vi "Get dBSPL from Frequency Amplitude List.vi"(0 "Semiconductor Module Context":T2, 5 "Sampling Rate":dbl format="%#_13g", 7 "Per Site Freq-Amp Data":T1[](array[typedef]), 11 "error in (no error)":errorcluster) -> (4 "Per-Site Per-FreqAmpPair dB SPL":dbl[][](array[numeric]), 15 "error out":errorcluster)   [LabVIEW 2020]
doc: "VI returns the Per-Site dB SPL value for Frequency-Amplitude List passed by user under specified sampling rate."
uses:
  <vilib>/NI_TestStand_SemiconductorModule/NI_TestStand_Semiconductor_Module.lvlibp/PinMap/General/SemiconductorModuleContext.ctl
  Per Site Sweep Data.ctl
  39a3ab5d-a6ea-4647-a559-e26a8959450b.vi
  6f0c4c81-6e94-4ac5-a946-327ae8ed193a.vi
  5552eb16-1d18-42dc-8af5-180ba06daae6.vi
  39a3ab5d-a6ea-4647-a559-e26a8959450b.vi/33b32ade-f888-404a-a29a-eab858b439c4.vi
  <vilib>/measure/matone.llb/Extract Single Tone Information N Chan.vi
  <vilib>/NI_TestStand_SemiconductorModule/NI_TestStand_Semiconductor_Module.lvlibp
  <vilib>/measure/NI_MAPro.lvlib
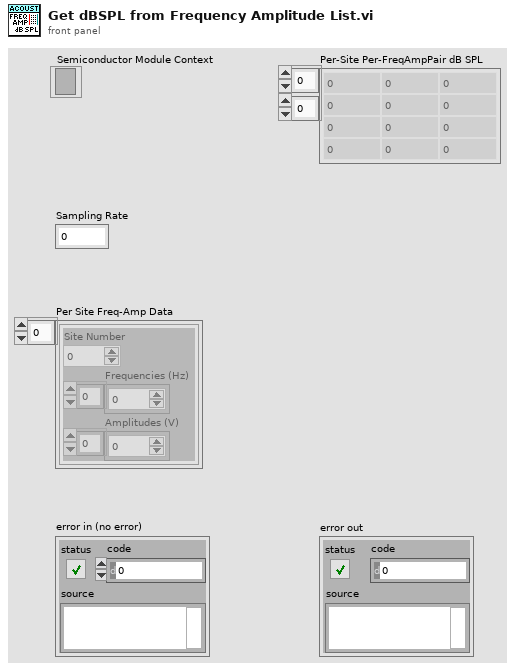
[diagram p1: front panel]
types:
  T1 = typedef "Per Site Sweep Data.ctl" = cluster{"Site Number":i32, "Frequencies (Hz)":dbl[], "Amplitudes (V)":dbl[]}
  T2 = typedef "NI_TestStand_Semiconductor_Module.lvlibp/SemiconductorModuleContext.ctl" = refnum<k7>
  T3 = typedef "TSM DAQmx Multi-Task.ctl" = cluster{"Pin Query Context":refnum<class "MultiplePinMultipleSessionQueryContext.lvclass">, "SSC":T4[], "Site Numbers":i32[], "Pins":tag[]}
  T4 = typedef "SSC DAQmx.ctl" = cluster{"DAQmx Task ":refnum<k21>, "Channels":string, "Channel Lists":string}
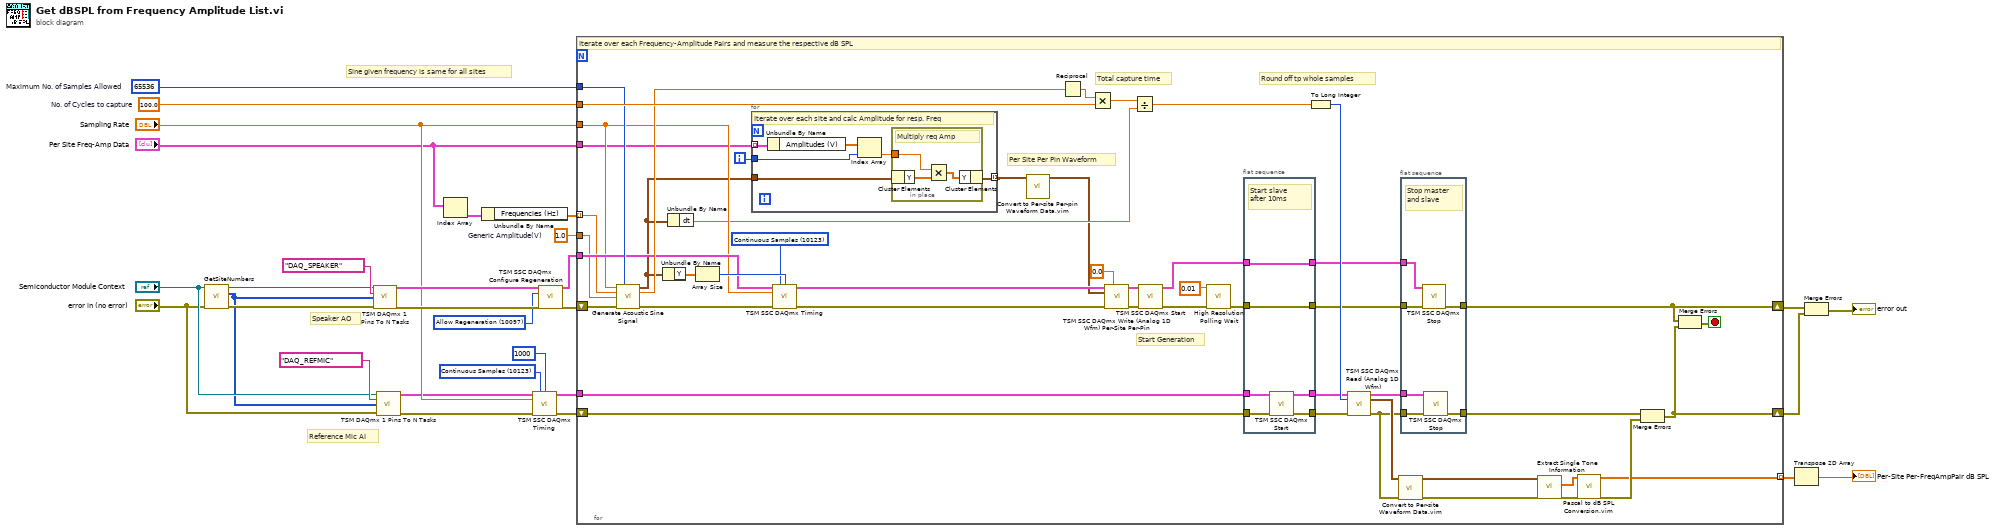
[diagram p0: block diagram]
diagram:
  w1 = 1.0  # Generic Amplitude(V)
  w11 = 65536  # Maximum No. of Samples Allowed
  w16 = 100.0  # No. of Cycles to capture
  w20 = 10123 items=["Finite Samples"=10178, "Continuous Samples"=10123, "Hardware Timed Single Point"=12522] ("Sample Mode")
  w27 = 10097 items=["Allow Regeneration"=10097, "Do Not Allow Regeneration"=10158] ("RegenMode")
  # "Sine given frequency is same for all sites"
  # "Reference Mic AI"
  # "Speaker AO"
  n1 = call <vilib>:"GetSiteNumbers.vi"("error in (no error)"="error in (no error)", "Semiconductor Module Context"="Semiconductor Module Context") -> ("error out"=w25:errorcluster, "Site Numbers"=w4:i32[], "Semiconductor Module Context Out"=w26:T2)  [unwired: 6 in, 1 out]
  n2 = call "TSM DAQmx 1 Pins To N Tasks.vi"("TSM context"=w26, "Pins"=tag "DAQ_SPEAKER", "Site Numbers"=w4, "error in"=w25) -> ("DAQ TSM Out"=w29:T3, "error out"=w30:errorcluster)  [unwired: 10 in]
  n3 = call "TSM DAQmx 1 Pins To N Tasks.vi"("TSM context"="Semiconductor Module Context", "Pins"=tag "DAQ_REFMIC", "Site Numbers"=w4, "error in"="error in (no error)") -> ("DAQ TSM Out"=w8:T3, "error out"=w9:errorcluster)  [unwired: 10 in]
  n4 = Index Array(array="Per Site Freq-Amp Data") -> (element=w3:T1)  [unwired: 1 in]
  n5 = Unbundle By Name(w3) -> ("Frequencies (Hz)"=w2:dbl[])
  n6 = call "TSM SSC DAQmx Timing.vi"("DAQ TSM in"=w8, "Sample Mode"=w20, "Samples"=1000, "Sample Rate"="Sampling Rate", "error in (no error)"=w9) -> ("DAQ TSM Out"=w19:T3, "error out"=w18:errorcluster)  [unwired: 9 in]
  n7 = call "TSM SSC DAQmx Configure Regeneration.vi"("TSM DAQmx In"=w29, "RegenMode"=w27, "error in (no error)"=w30) -> ("TSM DAQmx Out"=w24:T3, "error out"=w23:errorcluster)  [unwired: 11 in]
  n8 = for {
    shift-right: [w72] -> w15
    shift-left: w23 -> [w78]
    shift-right: [w71] -> w10
    shift-left: w18 -> [w75]
    tunnel: "Sampling Rate" -> [w62]
    tunnel: w16 -> [w77]
    tunnel: w11 -> [w76]
    tunnel: w24 -> [w64]
    tunnel: w19 -> [w74]
    tunnel: [w39] -> w7 mode=indexing
    tunnel: "Per Site Freq-Amp Data" -> [w36]
    tunnel: w2 -> [w37] mode=indexing
    tunnel: w1 -> [w38]
    i -> [w35]
    stop <- w70 stop-if-true
    w68 = 10123 items=["Finite Samples"=10178, "Continuous Samples"=10123, "Hardware Timed Single Point"=12522] ("Sample Mode")
    # "Per Site Per Pin Waveform"
    # "Start Generation"
    # "Round off tp whole samples"
    # "Total capture time"
    # "Iterate over each Frequency-Amplitude Pairs and measure the respective dB SPL"
    n9 = call "Generate Acoustic Sine Signal.vi"("Sampling Rate"=w62, "Maximum No. of Samples Allowed"=w76, "Frequency"=w37, "Sine wave amplitude"=w38, "error in (no error)"=w78) -> ("waveform"=w34:waveform(dbl), "Actual Frequency"=w73:dbl, "error out"=w67:errorcluster)  [unwired: 8 in]
    n10 = Unbundle By Name(w34) -> ("Y"=w65:dbl[])
    n11 = Unbundle By Name(w34) -> ("dt"=w44:dbl)
    n12 = Array Size(array=w65) -> (size(s)=w69:i32)
    n13 = for {
      tunnel: w36 -> [w84] mode=indexing
      tunnel: w35 -> [w82]
      tunnel: w34 -> [w81]
      tunnel: [w79] -> w33 mode=indexing
      # "Iterate over each site and calc Amplitude for resp. Freq"
      n14 = Unbundle By Name(w84) -> ("Amplitudes (V)"=w83:dbl[])
      n15 = Index Array(array=w83, index=w82) -> (element=w80:dbl)
      n16 = in-place {
        in-place-border: w80 -> [w86]
        # "Multiply req Amp"
        n17 = in-place-cluster #1(w81) -> ("Y"=w87:dbl[])
        n18 = Multiply(x=w86, y=w87) -> (x*y=w85:dbl[])
        n19 = in-place-cluster #1("Y"=w85) -> (w79:waveform(dbl))
      }
    }
    n20 = call "TSM SSC DAQmx Timing.vi"("DAQ TSM in"=w64, "Sample Mode"=w68, "Samples"=w69, "Sample Rate"=w62, "error in (no error)"=w67) -> ("DAQ TSM Out"=w63:T3, "error out"=w66:errorcluster)  [unwired: 9 in]
    n21 = call "Convert to Per-site Per-pin Waveform Data.vim"("Waveform In"=w33) -> ("Per Site Per Pin Waveform Out"=w32:waveform(dbl)[][])  [unwired: 14 in]
    n22 = Reciprocal(x=w73) -> (1/x=w43:dbl)
    n23 = Multiply(x=w43, y=w77) -> (x*y=w54:dbl)
    n24 = call "TSM SSC DAQmx Write (Analog 1D Wfm) Per-Site Per-Pin.vi"("DAQ TSM in"=w63, "Idle Channel Value (0)"=0.0, "Per-Site Per-Pin Waveforms in"=w32, "error in"=w66) -> ("DAQ TSM Out"=w61:T3, "error out"=w57:errorcluster)  [unwired: 10 in]
    n25 = Divide(x=w54, y=w44) -> (x/y=w53:dbl)
    n26 = call "TSM SSC DAQmx Start.vi"("TSM DAQmx In"=w61, "error in (no error)"=w57) -> ("TSM DAQmx Out"=w48:T3, "error out"=w55:errorcluster)  [unwired: 12 in]
    n27 = call <vilib>:"High Resolution Polling Wait.vi"("error in (no error)"=w55, "seconds to wait"=0.01) -> ("error out"=w46:errorcluster)  [unwired: 9 in]
    n28 = flat-sequence {
      tunnel: w75 -> [w93]
      tunnel: w74 -> [w92]
      tunnel: [w91] -> w50
      tunnel: [w90] -> w49
      tunnel: w48 -> [w89]
      tunnel: [w89] -> w47
      tunnel: w46 -> [w88]
      tunnel: [w88] -> w45
      frame #0 {
        # "Start slave after 10ms"
        n29 = call "TSM SSC DAQmx Start.vi"("TSM DAQmx In"=w92, "error in (no error)"=w93) -> ("TSM DAQmx Out"=w90:T3, "error out"=w91:errorcluster)  [unwired: 12 in]
      }
    }
    n30 = To Long Integer(number=w53) -> (32bit integer=w52:i32)
    n31 = call "TSM SSC DAQmx Read (Analog 1D Wfm).vi"("DAQ TSM in"=w49, "Samples to read"=w52, "error in"=w50) -> ("DAQ TSM Out"=w60:T3, "Per-Site Per-Pin Waveforms Out"=w59:waveform(dbl)[][], "error out"=w42:errorcluster)  [unwired: 10 in]
    n32 = call "Convert to Per-site Waveform Data.vim"("Per-Site Per-Pin Waveform In"=w59) -> ("Per-Site Waveform Out"=w58:waveform(dbl)[])  [unwired: 14 in]
    n33 = flat-sequence {
      tunnel: w45 -> [w99]
      tunnel: w47 -> [w98]
      tunnel: [w97] -> w72
      tunnel: w42 -> [w96]
      tunnel: [w95] -> w41
      tunnel: w60 -> [w94]
      frame #0 {
        # "Stop master and slave"
        n34 = call "TSM SSC DAQmx Stop.vi"("TSM DAQmx In"=w98, "error in (no error)"=w99) -> ("error out"=w97:errorcluster)  [unwired: 12 in, 1 out]
        n35 = call "TSM SSC DAQmx Stop.vi"("TSM DAQmx In"=w94, "error in (no error)"=w96) -> ("error out"=w95:errorcluster)  [unwired: 12 in, 1 out]
      }
    }
    n36 = call-poly <vilib>:"Extract Single Tone Information.vi"("error in (no error)"=w42, "time signals in"=w58) -> ("error out"=w40:errorcluster, "detected amplitudes"=w31:dbl[])  [unwired: 4 in, 4 out]
    n37 = call "Pascal to dB SPL Conversion.vim"("Pascals"=w31) -> ("dbSPL"=w39:dbl[])  [unwired: 14 in]
    n38 = Merge Errors(w41, w40) -> (w71:errorcluster)
    n39 = Merge Errors(w72, w71) -> (w70:errorcluster)
  }
  n40 = Transpose 2D Array(2D array=w7) -> (transposed array=→"Per-Site Per-FreqAmpPair dB SPL":dbl[][])
  n41 = Merge Errors(w15, w10) -> (→"error out":errorcluster)
